vi "Parse Numeric.vi"(8 "error in (no error)":errorcluster, 10 "Index In":i32, 11 "JSON String":string) -> (0 "error out":errorcluster, 2 "Index Out":i32, 3 "JSON Value out":refnum<class "JSON Value.lvclass">)   [LabVIEW 2016, in "JSON Value.lvclass"]
uses:
  JSON Value.lvclass
  subVIs/Errors.ctl
  New JSON Value/New JSON (Numeric).vi
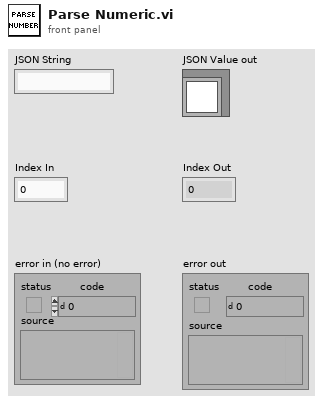
[diagram p1: front panel]
types:
  T1 = typedef "JSON Value.lvclass/Errors.ctl" = enum8{"No key", "Key path type", "Array OOB", "Type Mismatch", "Invalid Token"}
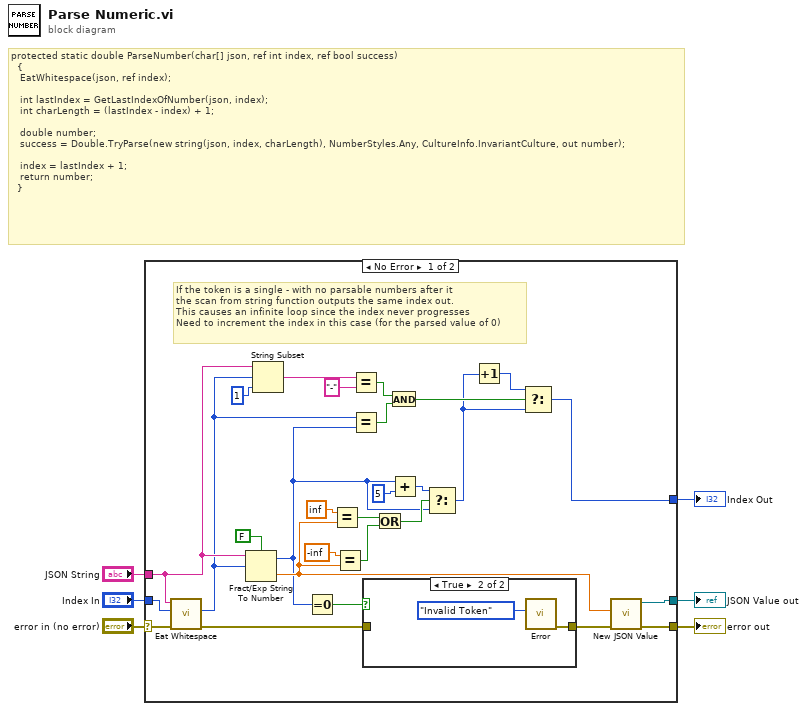
[diagram p0: block diagram]
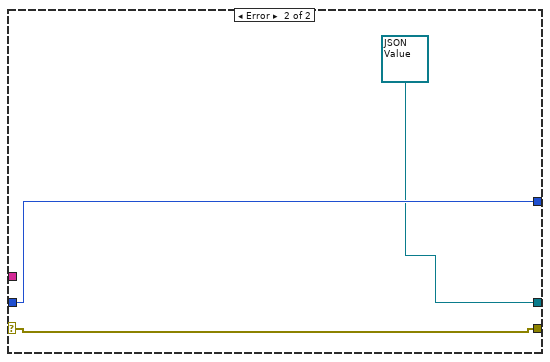
[diagram p3: hidden frame]
diagram:
  # "protected static double ParseNumber(char[] json, ref int index, ref bool success)\n\t\t{\n\t\t\tEatWhitespace(json, ref index);\n\n\t\t\tint lastIndex = GetLastIndexOfNumber(json, index);\n\t\t\tint charLength = (lastIndex - index) + 1;\n\n\t\t\tdouble number;\n\t\t\tsuccess = Double.TryParse(new string(json, index, charLength), NumberStyles.Any, CultureInfo.InvariantCulture, out number);\n\n\t\t\tindex = lastIndex + 1;\n\t\t\treturn number;\n\t\t}"
  n1 = case shown="No Error" "error in (no error)" {
    selector: "error in (no error)" -> [w33 w39]
    tunnel: [w32 w39] -> w5
    tunnel: [w31 refnum<class "JSON Value.lvclass"> refnum ("JSON out")] -> w1
    tunnel: "Index In" -> [w34 w40]
    tunnel: [w9 w40] -> w3
    tunnel: "JSON String" -> [w17 _]
    frame No Error {
      # "If the token is a single - with no parsable numbers after it\nthe scan from string function outputs the same index out.\nThis causes an infinite loop since the index never progresses\nNeed to increment the index in this case (for the parsed value of 0)"
      n2 = call "Eat Whitespace.vi"("error in (no error)"=w33, "Index In"=w34, "JSON String"=w17) -> ("error out"=w29:errorcluster, "Index Out"=w16:i32)  [unwired: 7 in]
      n3 = Fract/Exp String To Number(use system decimal point (T)=FALSE, string=w17, offset=w16) -> (offset past number=w18:i32, number=w23:dbl)  [unwired: 1 in]
      n4 = String Subset(string=w17, offset (0)=w16, length (rest)=1 ("length (rest)")) -> (substring=w14:string)
      n5 = Equal To 0?(x=w18) -> (x = 0?=w30:bool)
      n6 = Equal?(x=inf, y=w23) -> (x = y?=w25:bool)
      n7 = Equal?(x=-inf, y=w23) -> (x = y?=w22:bool)
      n8 = Equal?(x=w14, y="-") -> (x = y?=w12:bool)
      n9 = Equal?(x=w16, y=w18) -> (x = y?=w11:bool)
      n10 = case shown="True" w30 {
        tunnel: w29 -> [w35 _]
        tunnel: [w35 w37] -> w28
        frame False {
        }
        frame True {
          n11 = call "Error.vi"("Error"=Errors."Invalid Token") -> ("error out"=w37:errorcluster)  [unwired: 9 in]
        }
      }
      n12 = Or(x=w25, y=w22) -> (x .or. y?=w21:bool)
      n13 = And(x=w12, y=w11) -> (x .and. y?=w10:bool)
      n14 = Add(x=w18, y=5) -> (x+y=w19:i32)
      n15 = Select(t=w19, s=w21, f=w18) -> (s? t:f=w8:i32)
      n16 = Increment(x=w8) -> (x+1=w7:i32)
      n17 = Select(t=w7, s=w10, f=w8) -> (s? t:f=w9:i32)
      n18 = call-poly "New JSON Value.vi"("error in (no error)"=w28, "value"=w23) -> ("error out"=w32:errorcluster, "JSON Value out"=w31:refnum<class "JSON Value.lvclass">)  [unwired: 8 in]
    }
    frame Error {
    }
  }
  "error out" <- w5
  "Index Out" <- w3
  "JSON Value out" <- w1
